vi "reshapeINfo.vi"(10 "Clibration":T4={"cam 0"={"incident ANGLE COMPENSATION"=[], "dp/B [MeV/C/B]"=[], "charge compensation"=[], "Momentum [MeV/C]"=[], "energyDependence Input"=[], "pixel angle (y)"=[], "dp [MeV/C/] "=[], "angle 2Dfor spectrumj"=[], "dp [MeV/C] 2D"=[], "charge compensation 2D"=[], "Screen&Camera 2"={"Screen Orientation"="Regular", "Screen angle"="Flat", "Lens"=enum."FL1-f8x08", "Calibration (mm/pix)"=1.0}, "ROI info"={"npix-X"=0, "npix-Y"=0, "Left [pix]"=0.0, "Top [pix]"=0.0}, "Y 2D full angle"=[], "calib pixel"={"y1(pixel)"=[], "y2(pixel)"=[], "dp/B [MeV/C/B] (pixel)"=[], "energyDependence Input(pixel)"=[], "bending angle [deg](pixel)"=[], "total path(pixel)"=[], "pixel angle (y)(pixel)"=[], "energy dependence (pixel)"=[], "charge compensation (pixel)"=[], "Momentum [MeV/C](pixel)"=[], "angular compensation(pixel)"=[]}, "2D"={"dp"=[], "chargeCompensation"=[], "angle"=[], "Momentum"=[]}, "UserROI"={"Width"=0.0, "Hight"=0.0, "OffsetX"=0.0, "OffsetY"=0.0}, "final"={"X"=[], "xi"=[], "delta momentum"=0.0, "Y"=[], "yi"=[], "angle (Y)"=[], "delta angle"=0.0, "scale delta angle"=0.0, "intraX"=0.0, "intraY"=0.0, "mask"=[]}, "B[T]"=0.0, "index"=0.0}, "cam 1"={"incident ANGLE COMPENSATION"=[], "dp/B [MeV/C/B]"=[], "charge compensation"=[], "Momentum [MeV/C]"=[], "energyDependence Input"=[], "pixel angle (y)"=[], "dp [MeV/C/] "=[], "angle 2Dfor spectrumj"=[], "dp [MeV/C] 2D"=[], "charge compensation 2D"=[], "Screen&Camera 2"={"Screen Orientation"="Regular", "Screen angle"="Flat", "Lens"=enum."FL1-f8x08", "Calibration (mm/pix)"=1.0}, "ROI info"={"npix-X"=0, "npix-Y"=0, "Left [pix]"=0.0, "Top [pix]"=0.0}, "Y 2D full angle"=[], "calib pixel"={"y1(pixel)"=[], "y2(pixel)"=[], "dp/B [MeV/C/B] (pixel)"=[], "energyDependence Input(pixel)"=[], "bending angle [deg](pixel)"=[], "total path(pixel)"=[], "pixel angle (y)(pixel)"=[], "energy dependence (pixel)"=[], "charge compensation (pixel)"=[], "Momentum [MeV/C](pixel)"=[], "angular compensation(pixel)"=[]}, "2D"={"dp"=[], "chargeCompensation"=[], "angle"=[], "Momentum"=[]}, "UserROI"={"Width"=0.0, "Hight"=0.0, "OffsetX"=0.0, "OffsetY"=0.0}, "final"={"X"=[], "xi"=[], "delta momentum"=0.0, "Y"=[], "yi"=[], "angle (Y)"=[], "delta angle"=0.0, "scale delta angle"=0.0, "intraX"=0.0, "intraY"=0.0, "mask"=[]}, "B[T]"=0.0, "index"=0.0}, "cam 2"={"incident ANGLE COMPENSATION"=[], "dp/B [MeV/C/B]"=[], "charge compensation"=[], "Momentum [MeV/C]"=[], "energyDependence Input"=[], "pixel angle (y)"=[], "dp [MeV/C/] "=[], "angle 2Dfor spectrumj"=[], "dp [MeV/C] 2D"=[], "charge compensation 2D"=[], "Screen&Camera 2"={"Screen Orientation"="Regular", "Screen angle"="Flat", "Lens"=enum."FL1-f8x08", "Calibration (mm/pix)"=1.0}, "ROI info"={"npix-X"=0, "npix-Y"=0, "Left [pix]"=0.0, "Top [pix]"=0.0}, "Y 2D full angle"=[], "calib pixel"={"y1(pixel)"=[], "y2(pixel)"=[], "dp/B [MeV/C/B] (pixel)"=[], "energyDependence Input(pixel)"=[], "bending angle [deg](pixel)"=[], "total path(pixel)"=[], "pixel angle (y)(pixel)"=[], "energy dependence (pixel)"=[], "charge compensation (pixel)"=[], "Momentum [MeV/C](pixel)"=[], "angular compensation(pixel)"=[]}, "2D"={"dp"=[], "chargeCompensation"=[], "angle"=[], "Momentum"=[]}, "UserROI"={"Width"=0.0, "Hight"=0.0, "OffsetX"=0.0, "OffsetY"=0.0}, "final"={"X"=[], "xi"=[], "delta momentum"=0.0, "Y"=[], "yi"=[], "angle (Y)"=[], "delta angle"=0.0, "scale delta angle"=0.0, "intraX"=0.0, "intraY"=0.0, "mask"=[]}, "B[T]"=0.0, "index"=0.0}, "cam 3"={"incident ANGLE COMPENSATION"=[], "dp/B [MeV/C/B]"=[], "charge compensation"=[], "Momentum [MeV/C]"=[], "energyDependence Input"=[], "pixel angle (y)"=[], "dp [MeV/C/] "=[], "angle 2Dfor spectrumj"=[], "dp [MeV/C] 2D"=[], "charge compensation 2D"=[], "Screen&Camera 2"={"Screen Orientation"="Regular", "Screen angle"="Flat", "Lens"=enum."FL1-f8x08", "Calibration (mm/pix)"=1.0}, "ROI info"={"npix-X"=0, "npix-Y"=0, "Left [pix]"=0.0, "Top [pix]"=0.0}, "Y 2D full angle"=[], "calib pixel"={"y1(pixel)"=[], "y2(pixel)"=[], "dp/B [MeV/C/B] (pixel)"=[], "energyDependence Input(pixel)"=[], "bending angle [deg](pixel)"=[], "total path(pixel)"=[], "pixel angle (y)(pixel)"=[], "energy dependence (pixel)"=[], "charge compensation (pixel)"=[], "Momentum [MeV/C](pixel)"=[], "angular compensation(pixel)"=[]}, "2D"={"dp"=[], "chargeCompensation"=[], "angle"=[], "Momentum"=[]}, "UserROI"={"Width"=0.0, "Hight"=0.0, "OffsetX"=0.0, "OffsetY"=0.0}, "final"={"X"=[], "xi"=[], "delta momentum"=0.0, "Y"=[], "yi"=[], "angle (Y)"=[], "delta angle"=0.0, "scale delta angle"=0.0, "intraX"=0.0, "intraY"=0.0, "mask"=[]}, "B[T]"=0.0, "index"=0.0}}, 11 "Settings":T13) -> (2 "reshapeInfo out":T1)   [LabVIEW 2020]
uses:
  MagAnalysis_Online/settings_TypDef.ctl
  CamSettings_Typdef.ctl
  CamSettingSUB_TypDEf.ctl
  CamAndObj_TypDEf.ctl
  OnOffTypeDef.ctl
  userROI.ctl
  source/Device Drivers/shared/numericVariable_TypeDef.ctl
  CamRoiTypDef.ctl
  SrewMaster_TYpDef.ctl
  srew_TypDEf.ctl
  ScrewSub_Typdef.ctl
  screwstart.ctl
  Calib_Typdef.ctl
  calib_Sub_Typdef.ctl
  ScreenCam2_TypDEf.ctl
  ROIInfo_TypDef.ctl
  calibPixel.ctl
  2DTypDef.ctl
  finalCalibTypdef.ctl
  reshapeINfo_TypDef.ctl
  emptyArray_TYpDEf.ctl
  emptyArrayCamX_TypDef.ctl
  reshapeArrayCommand_TypDEf.ctl
  NI_AALBase.lvlib
  source/Device Drivers/BaseDriver/BaseDriver.lvclass
  MagAnalysis_Online.lvclass
panel:
  out "start Y":dbl[](array[numeric])
  out "element":dbl
  out "Numeric":i32
  out "XY Graph":cluster{"Y":dbl[], "Y":dbl[]}[](graph)
  out "Array 4":dbl[](array[numeric])
  out "total":i32[](array[numeric])
  out "higherBuffer":i32[](array[numeric])
  out "lowerBuffer":i32[](array[numeric])
  out "MINY":dbl[](array[numeric])
  out "MaxY":dbl[](array[numeric])
  out "x/y":dbl[](array[numeric])
  out "MinY":dbl[](array[numeric])
  out "Hight (ALL)":dbl
  out "delta Y":dbl[](array[numeric])
  out "minY":dbl
  out "maxY":dbl
  out "width":i32[](array[numeric])
  out "Hight":i32[](array[numeric])
  out "width?":dbl[](array[numeric])
  out "Array":dbl[](array[numeric])
  out "delta":dbl[](array[numeric])
  out "max":dbl[](array[numeric])
  out "min":dbl[](array[numeric])
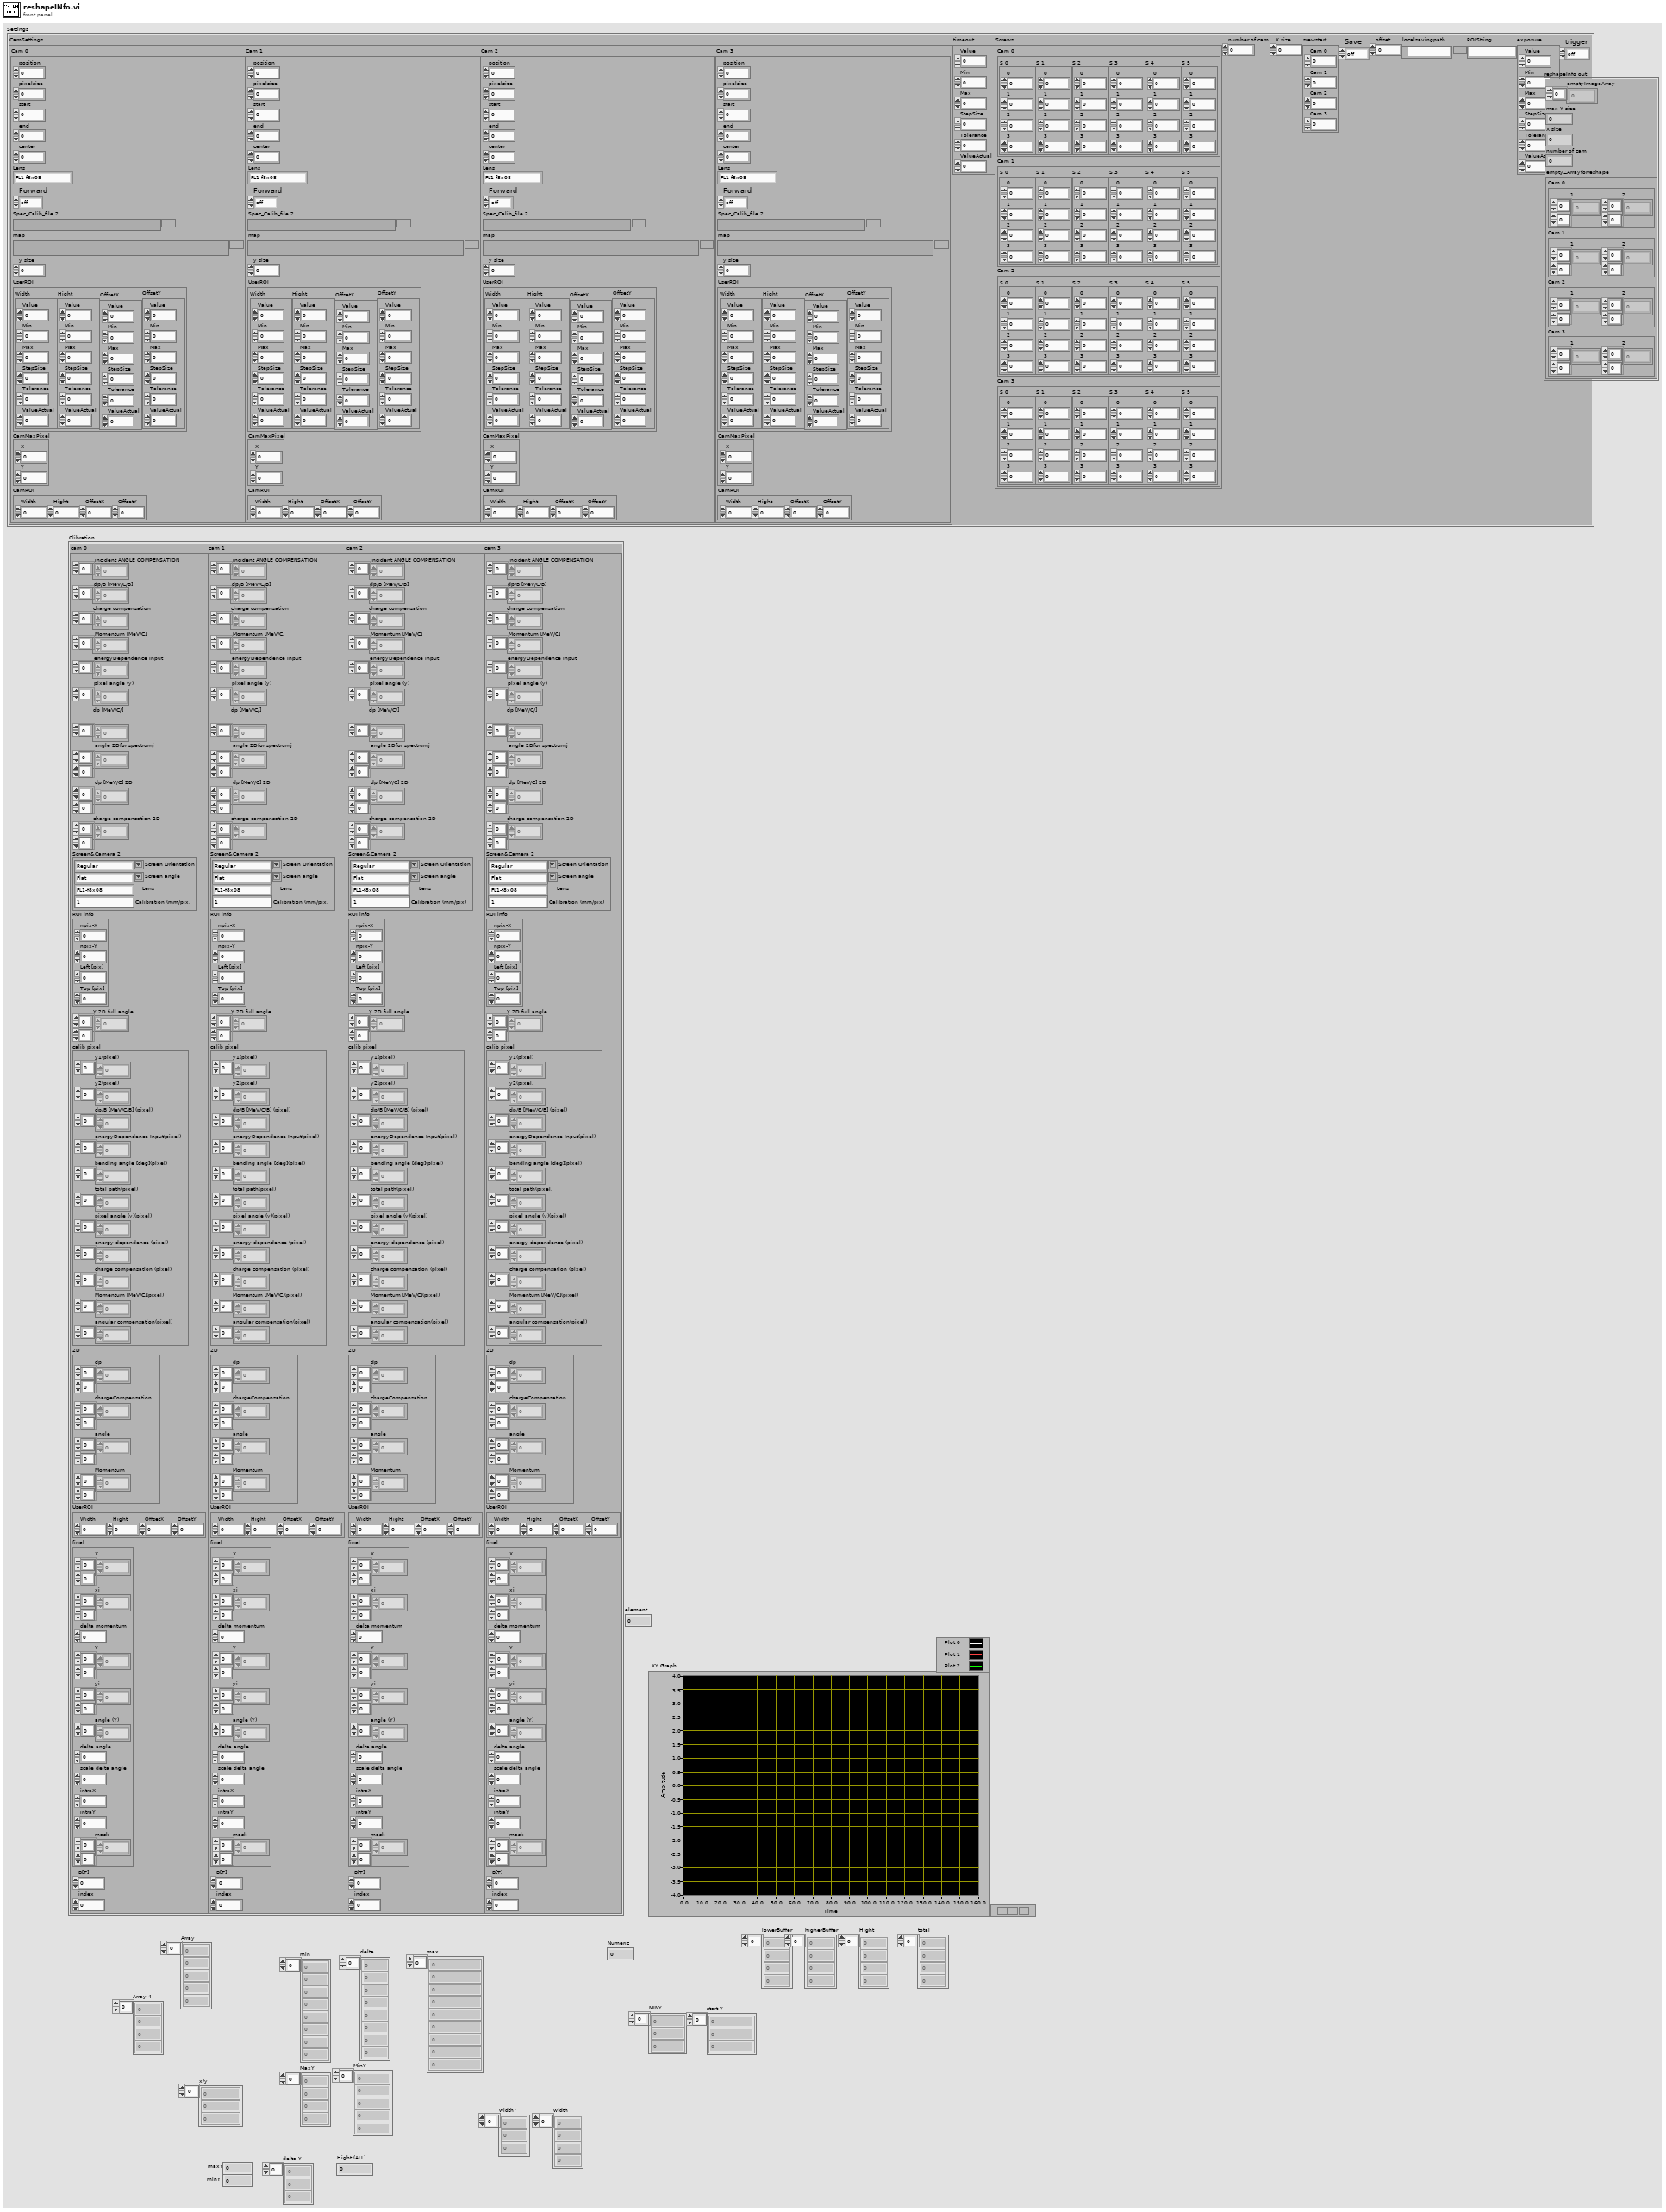
[diagram p1: front panel]
types:
  T1 = typedef "reshapeINfo_TypDef.ctl" = cluster{"emptyImageArray":dbl[], "max Y size":i32, "X size":i32, "number of cam":i32, "emptyZArrayforreshape":T2}
  T2 = typedef "emptyArray_TYpDEf.ctl" = cluster{"Cam 0":T3, "Cam 1":T3, "Cam 2":T3, "Cam 3":T3}
  T3 = typedef "emptyArrayCamX_TypDef.ctl" = cluster{"1":dbl[][], "2":dbl[][]}
  T4 = typedef "Calib_Typdef.ctl" = cluster{"cam 0":T5, "cam 1":T5, "cam 2":T5, "cam 3":T5}
  T5 = typedef "calib_Sub_Typdef.ctl" = cluster{"incident ANGLE COMPENSATION":dbl[], "dp/B [MeV/C/B]":dbl[], "charge compensation":dbl[], "Momentum [MeV/C]":dbl[], "energyDependence Input":dbl[], "pixel angle (y)":dbl[], "dp [MeV/C/] ":dbl[], "angle 2Dfor spectrumj":dbl[][], "dp [MeV/C] 2D":dbl[][], "charge compensation 2D":dbl[][], "Screen&Camera 2":T6, "ROI info":T8, "Y 2D full angle":dbl[][], "calib pixel":T9, "2D":T10, "UserROI":T11, "final":T12, "B[T]":dbl, "index":dbl}
  T6 = typedef "ScreenCam2_TypDEf.ctl" = cluster{"Screen Orientation":string, "Screen angle":string, "Lens":T7, "Calibration (mm/pix)":dbl}
  T7 = typedef "CamAndObj_TypDEf.ctl" = enum16{"FL1-f8x08", "FL1-f8x06", "FL1-f8", "ch300-f50", "FL2G-f8", "FL3M14-f8", "FL3M14-f8x08", "FL3M14-f8x08(2x2)"}
  T8 = typedef "ROIInfo_TypDef.ctl" = cluster{"npix-X":i32, "npix-Y":i32, "Left [pix]":dbl, "Top [pix]":dbl}
  T9 = typedef "calibPixel.ctl" = cluster{"y1(pixel)":dbl[], "y2(pixel)":dbl[], "dp/B [MeV/C/B] (pixel)":dbl[], "energyDependence Input(pixel)":dbl[], "bending angle [deg](pixel)":dbl[], "total path(pixel)":dbl[], "pixel angle (y)(pixel)":dbl[], "energy dependence (pixel)":dbl[], "charge compensation (pixel)":dbl[], "Momentum [MeV/C](pixel)":dbl[], "angular compensation(pixel)":dbl[]}
  T10 = typedef "2DTypDef.ctl" = cluster{"dp":dbl[][], "chargeCompensation":dbl[][], "angle":dbl[][], "Momentum":dbl[][]}
  T11 = typedef "CamRoiTypDef.ctl" = cluster{"Width":dbl, "Hight":dbl, "OffsetX":dbl, "OffsetY":dbl}
  T12 = typedef "finalCalibTypdef.ctl" = cluster{"X":dbl[][], "xi":dbl[][], "delta momentum":dbl, "Y":dbl[][], "yi":dbl[][], "angle (Y)":dbl[], "delta angle":dbl, "scale delta angle":dbl, "intraX":dbl, "intraY":dbl, "mask":dbl[][]}
  T13 = typedef "MagAnalysis_Online.lvclass/settings_TypDef.ctl" = cluster{"CamSettings":T14, "timeout":T18, "Screws":T19, "number of cam":dbl, "X size":dbl, "srewstart":T22, "Save":T16, "offset":dbl, "localsavingpath":path, "ROIString":string, "exposure":T18, "trigger":T16}
  T14 = typedef "CamSettings_Typdef.ctl" = cluster{"Cam 0":T15, "Cam 1":T15, "Cam 2":T15, "Cam 3":T15}
  T15 = typedef "CamSettingSUB_TypDEf.ctl" = cluster{"position":dbl, "pixelsize":dbl, "start":dbl, "end":dbl, "center":dbl, "Lens":T7, "Forward":T16, "Spec_Calib_file 2":path, "map":path, "y size":i32, "UserROI":T17, "CamMaxPixel":cluster{"X":i32, "Y":i32}, "CamROI":T11}
  T16 = typedef "OnOffTypeDef.ctl" = enum16{"off", "on"}
  T17 = typedef "userROI.ctl" = cluster{"Width":T18, "Hight":T18, "OffsetX":T18, "OffsetY":T18}
  T18 = typedef "BaseDriver.lvclass/numericVariable_TypeDef.ctl" = cluster{"Value":dbl, "Min":dbl, "Max":dbl, "StepSize":dbl, "Tolerance":dbl, "ValueActual":dbl}
  T19 = typedef "SrewMaster_TYpDef.ctl" = cluster{"Cam 0":T20, "Cam 1":T20, "Cam 2":T20, "Cam 3":T20}
  T20 = typedef "srew_TypDEf.ctl" = cluster{"S 0":T21, "S 1":T21, "S 2":T21, "S 3":T21, "S 4":T21, "S 5":T21}
  T21 = typedef "ScrewSub_Typdef.ctl" = cluster{"0":i32, "1":i32, "2":i32, "3":i32}
  T22 = typedef "screwstart.ctl" = cluster{"Cam 0":dbl, "Cam 1":dbl, "Cam 2":dbl, "Cam 3":dbl}
  T23 = typedef "reshapeArrayCommand_TypDEf.ctl" = enum16{"init array", "addImage", "read", "init resolution"}
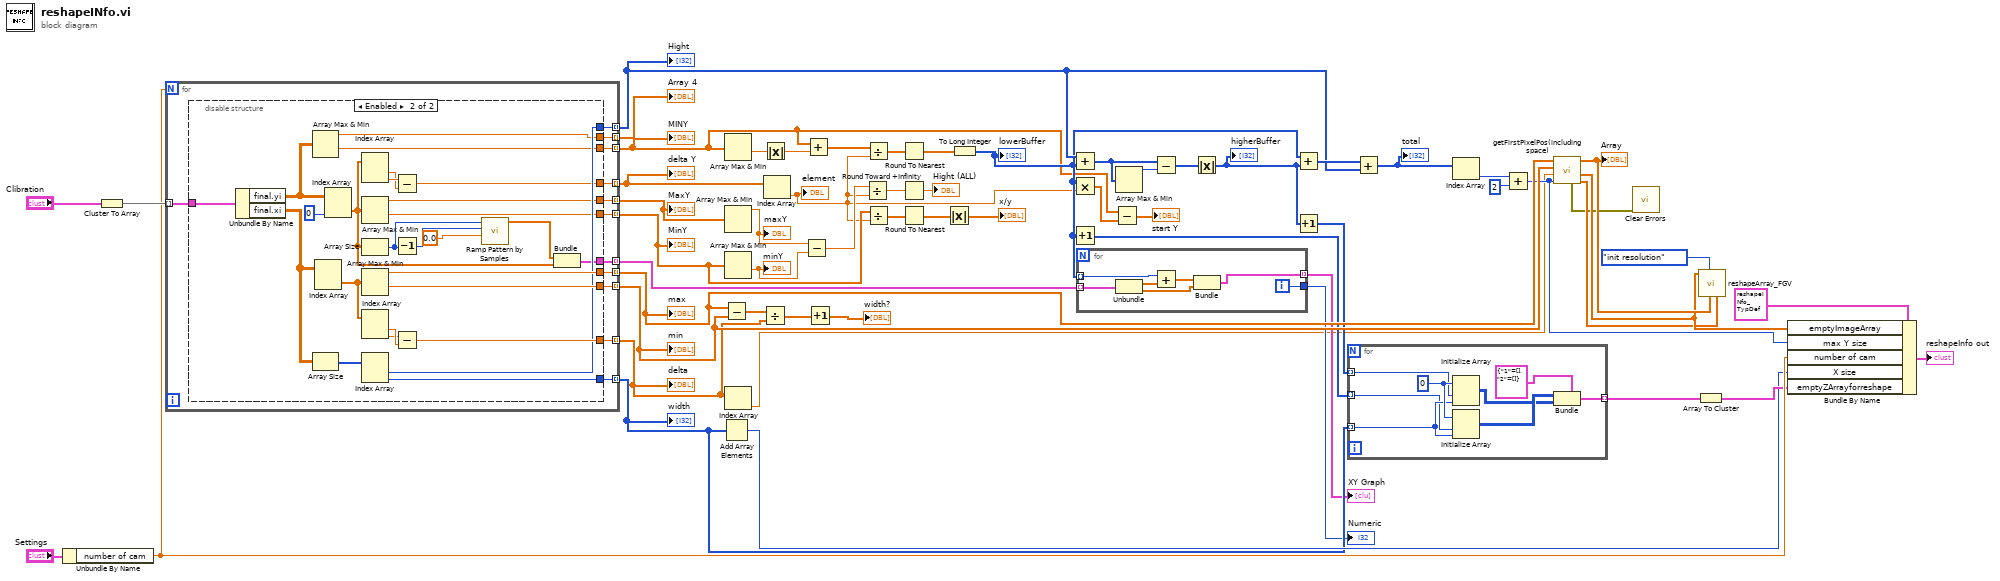
[diagram p0: block diagram]
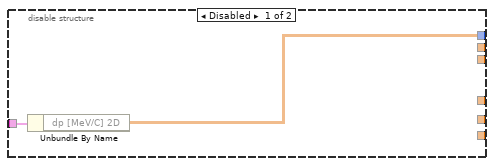
[diagram p2: hidden frame]
diagram:
  n1 = Unbundle By Name("Settings") -> ("number of cam"=w33:dbl)
  n2 = Cluster To Array(cluster="Clibration") -> (array=w57:T5[])
  n3 = for {
    N: w33 -> [_]
    tunnel: w57 -> [w71] mode=indexing
    tunnel: [w70] -> w29 mode=indexing
    tunnel: [w69] -> w52 mode=indexing
    tunnel: [w68] -> w51 mode=indexing
    tunnel: [w67] -> w50 mode=indexing
    tunnel: [w66] -> w21 mode=indexing
    tunnel: [w65] -> w38 mode=indexing
    tunnel: [w64] -> w34 mode=indexing
    tunnel: [w63] -> w41 mode=indexing
    tunnel: [w62] -> w4 mode=indexing
    tunnel: [w61] -> w31 mode=indexing
    tunnel: [w60] -> w13 mode=indexing
    n4 = disable-structure shown="Enabled" {
      disable-tunnel: w71 -> [w73 w99]
      disable-tunnel: [w72 w89] -> w70
      disable-tunnel: [_ w98] -> w69
      disable-tunnel: [_ w97] -> w68
      disable-tunnel: [_ w94] -> w67
      disable-tunnel: [_ w90] -> w66
      disable-tunnel: [_ w83] -> w65
      disable-tunnel: [_ w84] -> w64
      disable-tunnel: [_ w85] -> w63
      disable-tunnel: [_ w80] -> w62
      disable-tunnel: [_ w81] -> w61
      disable-tunnel: [_ w74] -> w60
      frame Disabled {
        n5 = Unbundle By Name(w73) -> ("dp [MeV/C] 2D"=w72:dbl[][])
      }
      frame Enabled {
        n6 = Unbundle By Name(w99) -> ("final.yi"=w82:dbl[][], "final.xi"=w92:dbl[][])
        n7 = Array Max & Min(array=w82) -> (max value=w81:dbl, min value=w80:dbl)  [unwired: 2 out]
        n8 = Array Size(array=w92) -> (size(s)=w91:i32[])
        n9 = Index Array(array=w92) -> (element=w93:dbl[])  [unwired: 2 in]
        n10 = Index Array(array=w82, index (col)=0 ("disabled index (col)")) -> (element=w75:dbl[])  [unwired: 1 in]
        n11 = Index Array(array=w75) -> (element #1=w86:dbl, element #2=w87:dbl)  [unwired: 2 in]
        n12 = Array Max & Min(array=w75) -> (max value=w83:dbl, min value=w84:dbl)  [unwired: 2 out]
        n13 = Array Size(array=w75) -> (size(s)=w78:i32)
        n14 = Array Max & Min(array=w93) -> (max value=w98:dbl, min value=w97:dbl)  [unwired: 2 out]
        n15 = Index Array(array=w93) -> (element #1=w96:dbl, element #2=w95:dbl)  [unwired: 2 in]
        n16 = Index Array(array=w91) -> (element #1=w89:i32, element #2=w90:i32)  [unwired: 2 in]
        n17 = Subtract(x=w87, y=w86) -> (x-y=w85:dbl)
        n18 = Decrement(x=w78) -> (x-1=w77:i32)
        n19 = Subtract(x=w95, y=w96) -> (x-y=w94:dbl)
        n20 = call "Ramp Pattern by Samples.vi"("start"=0.0 ("delta"), "end"=w77, "samples"=w78) -> ("Ramp Pattern"=w76:dbl[])  [unwired: 7 in, 1 out]
        n21 = Bundle("Ramp Pattern"=w76, "yi"=w75) -> (w74:cluster{"Ramp Pattern":dbl[], "yi":dbl[]})  [unwired: 1 in]
      }
    }
  }
  "min" <- w51
  "max" <- w52
  "delta" <- w50
  "Hight" <- w29
  "width" <- w21
  "delta Y" <- w41
  "MinY" <- w34
  "MaxY" <- w38
  "MINY" <- w4
  "Array 4" <- w31
  n22 = Subtract(x=w52, y=w51) -> (x-y=w53:dbl[])
  n23 = Add Array Elements(numeric array=w21) -> (sum=w22:i32)
  n24 = Array Max & Min(array=w4) -> (min value=w11:dbl)  [unwired: 3 out]
  n25 = Array Max & Min(array=w38) -> (max value=w44:dbl)  [unwired: 3 out]
  "maxY" <- w44
  n26 = Array Max & Min(array=w34) -> (min value=w43:dbl)  [unwired: 3 out]
  "minY" <- w43
  n27 = Index Array(array=w50) -> (element=w9:dbl)  [unwired: 1 in]
  n28 = Divide(x=w53, y=w50) -> (x/y=w46:dbl[])
  n29 = Absolute Value(x=w11) -> (abs(x)=w10:dbl)
  n30 = Index Array(array=w41) -> (element=w5:dbl)  [unwired: 1 in]
  "element" <- w5
  n31 = Subtract(x=w44, y=w43) -> (x-y=w42:dbl)
  n32 = Add(x=w4, y=w10) -> (x+y=w8:dbl[])
  n33 = Increment(x=w46) -> (x+1=→"width?":dbl[])
  n34 = Divide(x=w42, y=w5) -> (x/y=w40:dbl)
  n35 = Divide(x=w8, y=w5) -> (x/y=w7:dbl[])
  n36 = Divide(x=w34, y=w5) -> (x/y=w37:dbl[])
  n37 = Round To Nearest(number=w7) -> (nearest integer value=w32:dbl[])
  n38 = Round Toward +Infinity(x=w40) -> (ceil(x): smallest int >= x=→"Hight (ALL)":dbl)
  n39 = Round To Nearest(number=w37) -> (nearest integer value=w36:dbl[])
  n40 = Absolute Value(x=w36) -> (abs(x)=→"x/y":dbl[])
  n41 = To Long Integer(number=w32) -> (32bit integer=w6:i32[])
  "lowerBuffer" <- w6
  n42 = Add(x=w29, y=w6) -> (x+y=w28:i32[])
  n43 = Multiply(x=w6, y=w5) -> (x*y=w3:dbl[])
  n44 = Increment(x=w6) -> (x+1=w18:i32[])
  n45 = for {
    tunnel: [w106] -> w12 mode=indexing
    tunnel: [w105] -> w14
    tunnel: w13 -> [w104] mode=indexing
    tunnel: w6 -> [w100] mode=indexing
    i -> [w105]
    n46 = Unbundle(w104) -> ("Ramp Pattern"=w103:dbl[], "yi"=w101:dbl[])
    n47 = Add(x=w100, y=w103) -> (x+y=w102:dbl[])
    n48 = Bundle(w102, "yi"=w101) -> (w106:cluster{dbl[], "yi":dbl[]})  [unwired: 1 in]
  }
  "XY Graph" <- w12
  "Numeric" <- w14
  n49 = Subtract(x=w4, y=w3) -> (x-y=→"start Y":dbl[])
  n50 = Array Max & Min(array=w28) -> (max value=w27:i32)  [unwired: 3 out]
  n51 = Subtract(x=w28, y=w27) -> (x-y=w26:i32[])
  n52 = Absolute Value(x=w26) -> (abs(x)=w20:i32[])
  "higherBuffer" <- w20
  n53 = Add(x=w6, y=w20) -> (x+y=w30:i32[])
  n54 = Increment(x=w20) -> (x+1=w19:i32[])
  n55 = for {
    tunnel: w21 -> [w112] mode=indexing
    tunnel: w18 -> [w111] mode=indexing
    tunnel: [w110] -> w24 mode=indexing
    tunnel: w19 -> [w109] mode=indexing
    w113 = 0
    n56 = Initialize Array(w113, w109, w112) -> (w107:i32[][])
    n57 = Initialize Array(w113, w111, w112) -> (w108:i32[][])
    n58 = Bundle(cluster=T3 {"1"=[], "2"=[]} ("Cam 1"), "1"=w108, "2"=w107) -> (w110:T3)
  }
  n59 = Add(x=w30, y=w29) -> (x+y=w25:i32[])
  "total" <- w25
  n60 = Index Array(array=w25) -> (element=w17:i32)  [unwired: 1 in]
  n61 = Add(x=w17, y=2) -> (x+y=w15:i32)
  n62 = call "getFirstPixelPos(includingspace).vi"("y"=w15, "delta"=w9, "min"=w51, "max"=w52) -> ("delete"=w47:dbl[], "initialized array"=w48:dbl[], "position"=w49:dbl[], "error out"=w1:errorcluster)  [unwired: 3 in, 1 out]
  "Array" <- w49
  n63 = call "Clear Errors.vi"("error in (no error)"=w1) -> ()  [unwired: 5 in, 2 out]
  n64 = Array To Cluster(array=w24) -> (cluster=w23:cluster{"[0]":T3, "[1]":T3, "[2]":T3, "[3]":T3})
  n65 = call "reshapeArray_FGV.vi"("delete"=w47, "firstpixelpos"=w49, "command"=reshapeArrayCommand_TypDEf."init resolution", "emptyImageArray"=w48) -> ()  [unwired: 6 in, 2 out]
  n66 = Bundle By Name(cluster=T1 {"emptyImageArray"=[], "max Y size"=0, "X size"=0, "number of cam"=0, "emptyZArrayforreshape"={"Cam 0"={"1"=[], "2"=[]}, "Cam 1"={"1"=[], "2"=[]}, "Cam 2"={"1"=[], "2"=[]}, "Cam 3"={"1"=[], "2"=[]}}} ("reshapeInfo in"), "emptyImageArray"=w48, "max Y size"=w15, "number of cam"=w33, "X size"=w22, "emptyZArrayforreshape"=w23) -> (→"reshapeInfo out":T1)
